vi "shift visible array up four.vi"(8 "error in (no error)":errorcluster, 11 "Array in":refnum<vi>) -> (0 "error out":errorcluster, 3 "Array out":refnum<vi>)   [LabVIEW 2014, in "Tagbus PID Module editor node.lvclass"]
uses:
  Tagbus PID Module editor node.lvclass
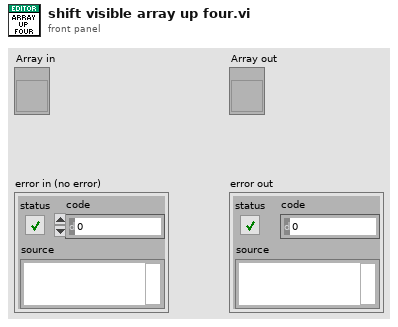
[diagram p1: front panel]
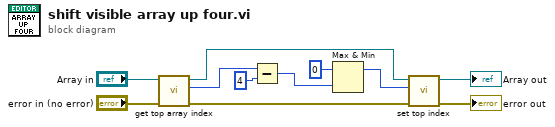
[diagram p0: block diagram]
diagram:
  n1 = call "get top array index.vi"("error in (no error)"="error in (no error)", "Array in"="Array in") -> ("error out"=w2:errorcluster, "top index"=w3:u32, "Array out"=w6:refnum<vi>)  [unwired: 6 in, 1 out]
  n2 = Subtract(x=w3, y=u32 4) -> (x-y=w10:u32)
  n3 = Max & Min(x=u32 0, y=w10) -> (max(x,y)=w1:u32)  [unwired: 1 out]
  n4 = call "set top index.vi"("error in (no error)"=w2, "Numeric"=w1, "Array in"=w6) -> ("error out"=→"error out":errorcluster, "Array out"=→"Array out":refnum<vi>)  [unwired: 7 in]
